vi "GPSMOTOR.vi"(0 "PastLat":dbl, 1 "PastLon":dbl, 2 "CurrentLat":dbl, 3 "CurrentLon":dbl, 4 "TargetLong":dbl, 5 "TargetLat":dbl, 6 "LeftIN":i8, 7 "RightIN":i8) -> (20 "LeftOUT":i8, 22 "RightOUT":i8)   [LabVIEW 2017]
panel:
  # "This vi handles the decision making based on current, past and target GPS data.\nIts ouput is the motor control values that will produce the desired behavior."
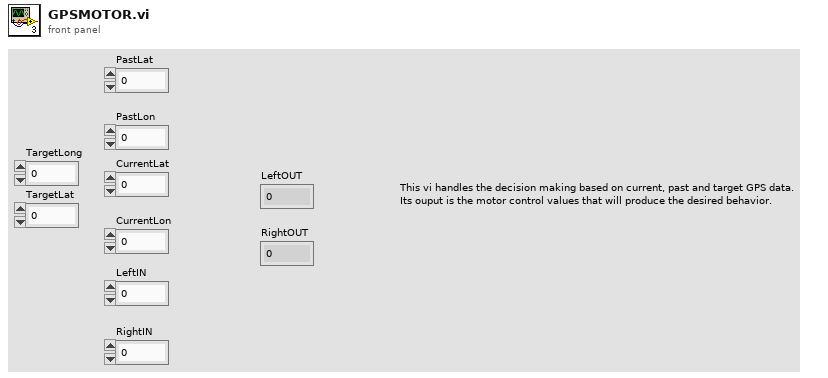
[diagram p1: front panel]
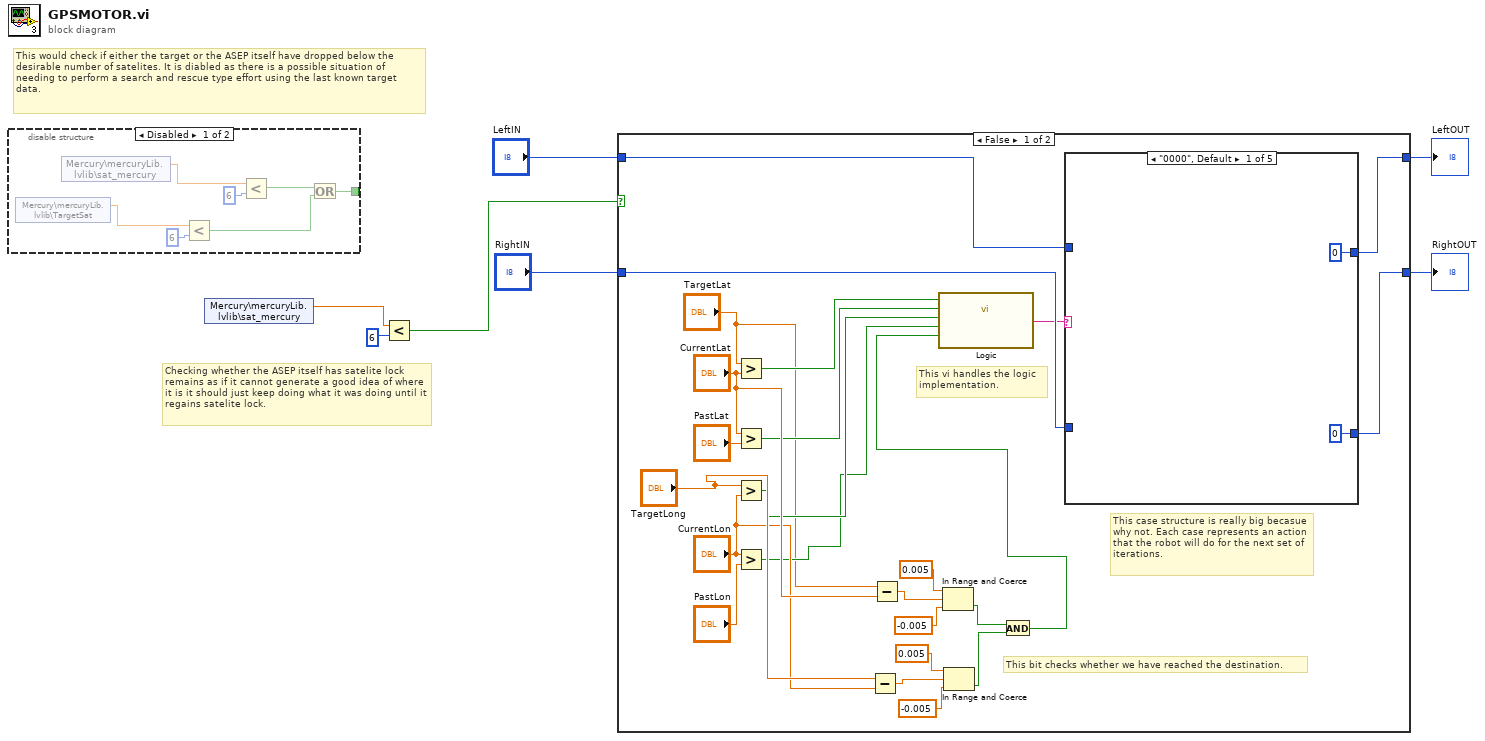
[diagram p0: block diagram]
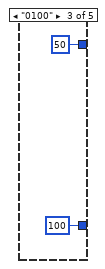
[diagram p4: hidden frame]
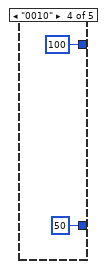
[diagram p5: hidden frame]
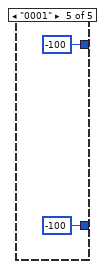
[diagram p6: hidden frame]
diagram:
  # "Checking whether the ASEP itself has satelite lock remains as if it cannot generate a good idea of where it is it should just keep doing what it was doing until it regains satelite lock."
  # "This would check if either the target or the ASEP itself have dropped below the desirable number of satelites. It is diabled as there is a possible situation of needing to perform a search and rescue type effort using the last known target data."
  n1 = disable-structure shown="Disabled" {
    disable-tunnel: [w13 _] -> _
    frame Disabled {
      n2 = shared-variable "Mercury\\mercuryLib.lvlib\\TargetSat"() -> (w9:dbl)  [unwired: 1 in, 1 out]
      n3 = shared-variable "Mercury\\mercuryLib.lvlib\\sat_mercury"() -> (w8:dbl)  [unwired: 1 in, 1 out]
      n4 = Less?(x=w9, y=6) -> (x < y?=w10:bool)
      n5 = Less?(x=w8, y=6) -> (x < y?=w12:bool)
      n6 = Or(x=w12, y=w10) -> (x .or. y?=w13:bool)
    }
    frame Enabled {
    }
  }
  n7 = shared-variable "Mercury\\mercuryLib.lvlib\\sat_mercury"() -> (w1:dbl)  [unwired: 1 in, 1 out]
  n8 = Less?(x=w1, y=6) -> (x < y?=w3:bool)
  n9 = case shown="False" w3 {
    tunnel: [w36 w50] -> w7
    tunnel: [w34 w49] -> w6
    tunnel: "LeftIN" -> [w35 w50]
    tunnel: "RightIN" -> [w33 w49]
    frame False {
      # "This case structure is really big becasue why not. Each case represents an action that the robot will do for the next set of iterations."
      # "This vi handles the logic\nimplementation."
      # "This bit checks whether we have reached the destination."
      n10 = Greater?(x="TargetLat", y="CurrentLat") -> (0:w22:bool)
      n11 = Greater?(x="CurrentLat", y="PastLat") -> (0:w21:bool)
      n12 = Greater?(x="TargetLong", y="CurrentLon") -> (0:w20:bool)
      n13 = Greater?(x="CurrentLon", y="PastLon") -> (0:w19:bool)
      n14 = Subtract(x="TargetLong", y="CurrentLon") -> (x-y=w16:dbl)
      n15 = Subtract(x="TargetLat", y="CurrentLat") -> (x-y=w17:dbl)
      n16 = In Range and Coerce(upper limit=0.005, x=w17, lower limit=-0.005) -> (In Range?=w32:bool)  [unwired: 1 out]
      n17 = In Range and Coerce(upper limit=0.005, x=w16, lower limit=-0.005) -> (In Range?=w27:bool)  [unwired: 1 out]
      n18 = And(x=w32, y=w27) -> (x .and. y?=w18:bool)
      n19 = call "Logic.vi"("DestinationReached"=w18, "D"=w19, "C"=w20, "B"=w21, "A"=w22) -> ("State"=w26:string)  [unwired: 6 in]
      n20 = case shown="\"0000\", Default" w26 {
        tunnel: [i8 0 ("LeftIN") w42 i8 50 ("LeftIN") i8 100 ("LeftIN") i8 -100 ("LeftIN")] -> w36
        tunnel: w35 -> [_ w42 _ _ _]
        tunnel: [i8 0 ("RightIN") w41 i8 100 ("RightIN") i8 50 ("RightIN") i8 -100 ("RightIN")] -> w34
        tunnel: w33 -> [_ w41 _ _ _]
        frame "0000", Default {
        }
        frame "1000" {
        }
        frame "0100" {
        }
        frame "0010" {
        }
        frame "0001" {
        }
      }
    }
    frame True {
    }
  }
  "RightOUT" <- w6
  "LeftOUT" <- w7
